vi "2019indicator.vi"() -> ()   [LabVIEW 2018]
panel:
  in  "stop":bool
  in  "Numeric":u16 max=4
  out "Ring":u16(ring)
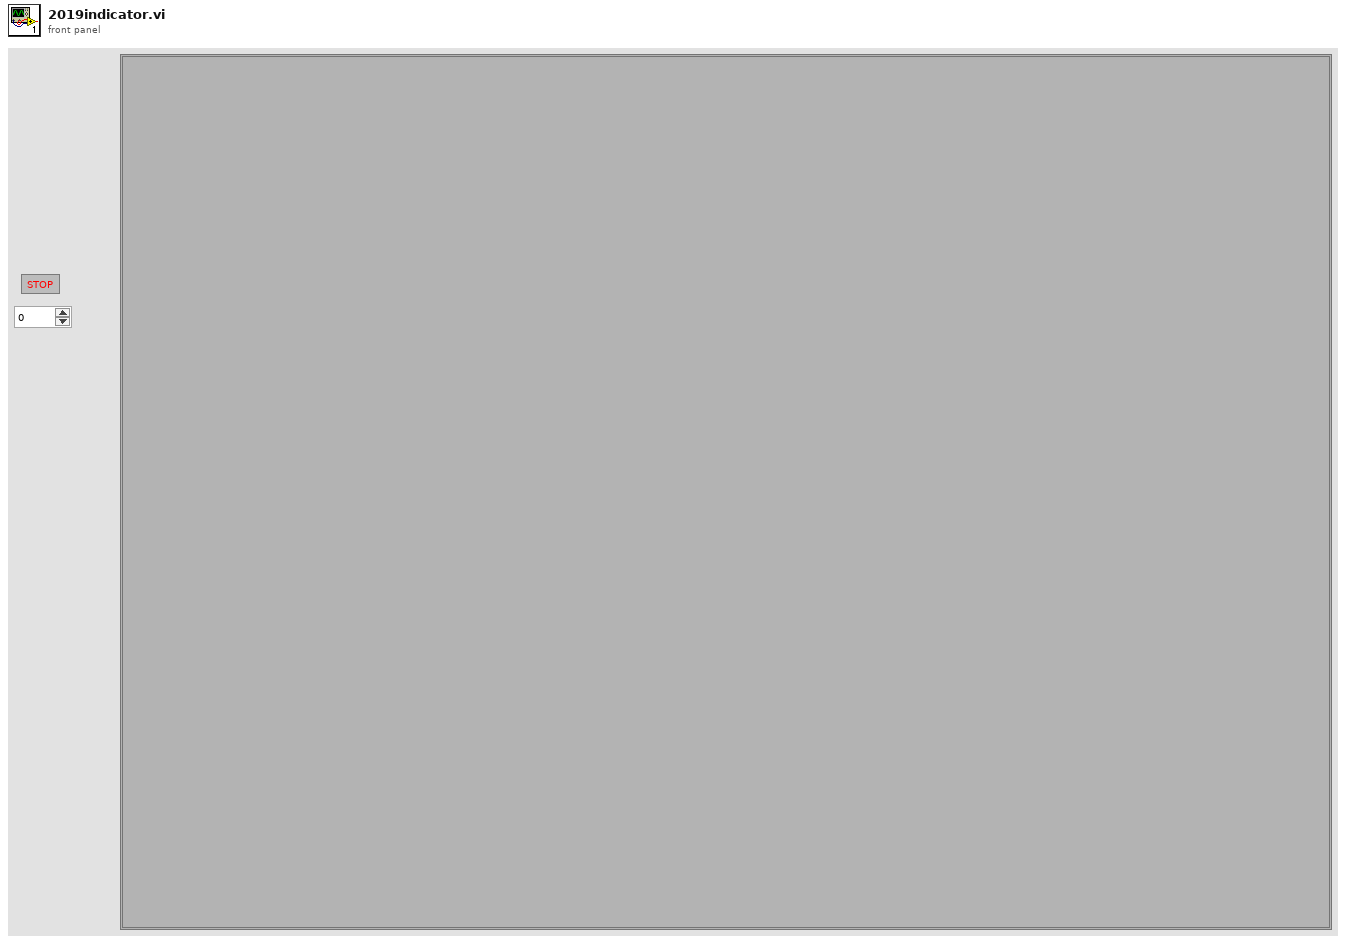
[diagram p1: front panel]
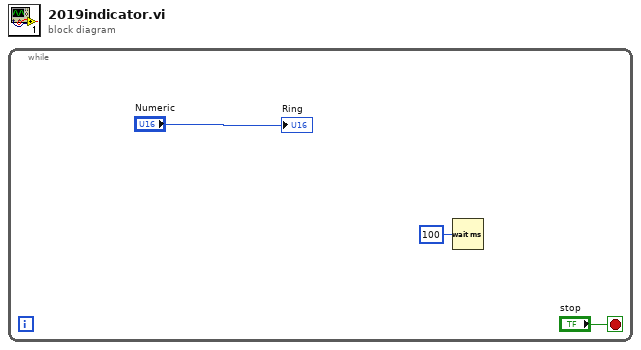
[diagram p0: block diagram]
diagram:
  n1 = while {
    stop <- "stop" stop-if-true
    n2 = Wait (ms)(milliseconds to wait=u32 100) -> ()  [unwired: 1 out]
    "Ring" <- "Numeric"
  }
